vi "@destroy.vi"(8 "error in (no error)":errorcluster, 11 "dotnet_system_exec in":refnum<class "dotnet_system_exec.lvclass">) -> (0 "error out":errorcluster, 3 "dotnet_system_exec out":refnum<class "dotnet_system_exec.lvclass">)   [LabVIEW 2015, in "dotnet_system_exec.lvclass"]
doc: "Stops the .NET System Process and destroy the necessary references."
uses:
  dotnet_system_exec.lvclass
  dotnet_system_exec.lvclass/dotnet_system_exec.ctl
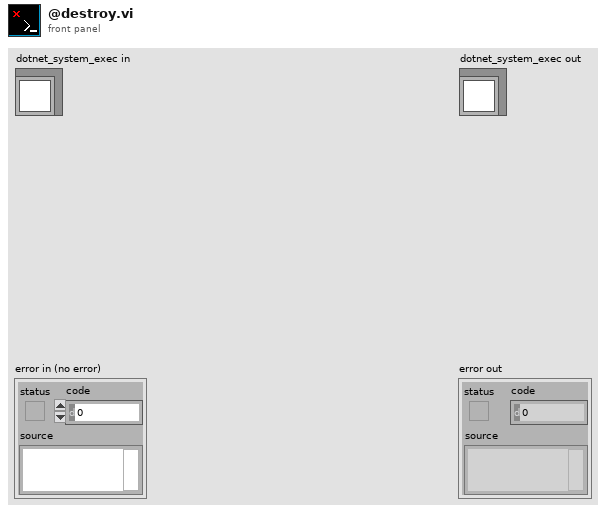
[diagram p1: front panel]
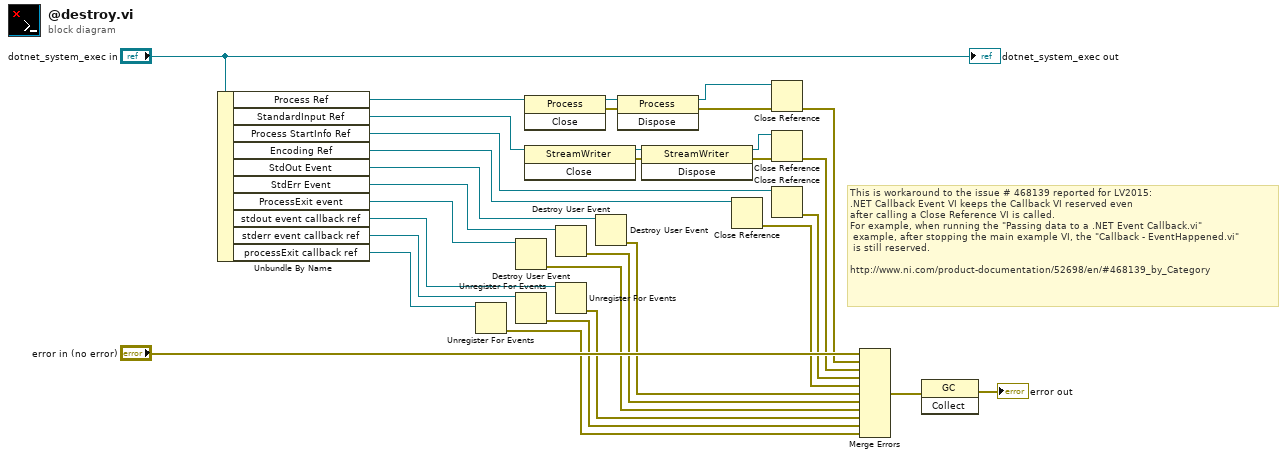
[diagram p0: block diagram]
diagram:
  # "This is workaround to the issue # 468139 reported for LV2015:\n.NET Callback Event VI keeps the Callback VI reserved even \nafter calling a Close Reference VI is called.\nFor example, when running the \"Passing data to a .NET Event Callback.vi\"\n example, after stopping the main example VI, the \"Callback - EventHappened.vi\"\n is still reserved.\n\nhttp://www.ni.com/product-documentation/52698/en/#468139_by_Category"
  n1 = Unbundle By Name("dotnet_system_exec in") -> ("Process Ref"=w10:refnum<k24>, "StandardInput Ref"=w21:refnum<k24>, "Process StartInfo Ref"=w20:refnum<k24>, "Encoding Ref"=w2:refnum<k24>, "StdOut Event"=w18:refnum<user-event>, "StdErr Event"=w17:refnum<user-event>, "ProcessExit event"=w5:refnum<user-event>, "stdout event callback ref"=w14:refnum<k27>, "stderr event callback ref"=w13:refnum<k27>, "processExit callback ref"=w6:refnum<k27>)
  n2 = Unregister For Events(event registration refnum=w6) -> (error out=w3:errorcluster)  [unwired: 1 in]
  n3 = Destroy User Event(user event=w5) -> (error out=w4:errorcluster)  [unwired: 1 in]
  n4 = Unregister For Events(event registration refnum=w13) -> (error out=w11:errorcluster)  [unwired: 1 in]
  n5 = invoke class="Process" method="Close"(reference=w10) -> (reference out=w26:refnum<k24>, error out=w25:errorcluster)  [unwired: 2 in, 1 out]
  n6 = invoke class="StreamWriter" method="Close"(reference=w21) -> (reference out=w30:refnum<k24>, error out=w29:errorcluster)  [unwired: 2 in, 1 out]
  n7 = Destroy User Event(user event=w17) -> (error out=w15:errorcluster)  [unwired: 1 in]
  n8 = Unregister For Events(event registration refnum=w14) -> (error out=w12:errorcluster)  [unwired: 1 in]
  n9 = Destroy User Event(user event=w18) -> (error out=w16:errorcluster)  [unwired: 1 in]
  n10 = invoke class="Process" method="Dispose"(reference=w26, error in=w25) -> (reference out=w23:refnum<k24>, error out=w24:errorcluster)  [unwired: 1 in, 1 out]
  n11 = invoke class="StreamWriter" method="Dispose"(reference=w30, error in=w29) -> (reference out=w27:refnum<k24>, error out=w28:errorcluster)  [unwired: 1 in, 1 out]
  n12 = Close Reference(reference=w2) -> (error out=w1:errorcluster)  [unwired: 1 in]
  n13 = Close Reference(reference=w23, error in (no error)=w24) -> (error out=w9:errorcluster)
  n14 = Close Reference(reference=w27, error in (no error)=w28) -> (error out=w22:errorcluster)
  n15 = Close Reference(reference=w20) -> (error out=w19:errorcluster)  [unwired: 1 in]
  n16 = Merge Errors("error in (no error)", w9, w22, w19, w1, w16, w15, w4, w12, w11, w3) -> (w8:errorcluster)
  n17 = invoke class="GC" method="Collect"(error in=w8) -> (error out=→"error out":errorcluster)  [unwired: 2 in, 2 out]
  "dotnet_system_exec out" <- "dotnet_system_exec in"
